vi "rad_Modify and Deploy RT-INI.vi"(5 "password":string, 7 "user (admin)":string="admin", 8 "error in (no error)":errorcluster, 9 "Run at Startup?":bool, 10 "Target settings":T1={"Hostname"="", "Serial number"="", "Product name"="", "Product code"=0, "System status"="", "Credential type"=enum."None/Unlocked", "User added?"=FALSE, "Primary NIC"={"MAC address"="", "IP Address Request Mode"=2, "IP address"="", "Subnet mask"="", "Gateway"="", "DNS server"=""}, "Real-Time CPU?"=FALSE} {"Primary NIC"."IP Address Request Mode" items=["Static"=1, "DHCP/Link-Local"=2, "Link-Local Only"=4, "DHCP Only"=8]}, 11 "temp folder":path) -> (0 "error out":errorcluster)   [LabVIEW 2018]
uses:
  Targets/TypeDefs/rad_Target Information.ctl
  Targets/TypeDefs/rad_Target Network Settings.ctl
  rad_Globals.vi
  <vilib>/Utility/config.llb/Write Key (Boolean).vi
  <vilib>/nisyscfg/Save Changes (Hardware).vi
  <vilib>/nisyscfg/Close (Hardware).vi
  <vilib>/nisyscfg/Close (System).vi
  <vilib>/Utility/config.llb/NI_LVConfig.lvlib
  <resource>/objmgr/motionsysapi.rc
  <resource>/objmgr/nisysapi.rc
  <vilib>/nisyscfg/nisyscfg.lvlib
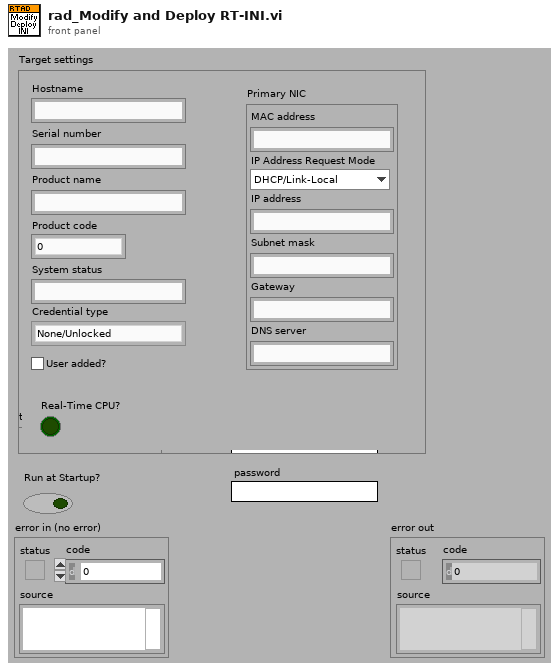
[diagram p1: front panel]
types:
  T1 = typedef "rad_Target Information.ctl" = cluster{"Hostname":string, "Serial number":string, "Product name":string, "Product code":i32, "System status":string, "Credential type":enum16{"None/Unlocked", "FTP Password", "NIAuth Credentials"}, "User added?":bool, "Primary NIC":T2, "Real-Time CPU?":bool}
  T2 = typedef "rad_Target Network Settings.ctl" = cluster{"MAC address":string, "IP Address Request Mode":i32, "IP address":string, "Subnet mask":string, "Gateway":string, "DNS server":string}
  T3 = enum16{"None/Unlocked", "FTP Password", "NIAuth Credentials"}
  T4 = typedef "NI_LVConfig.lvlib/Config Data RefNum.ctl" = refnum<k1>
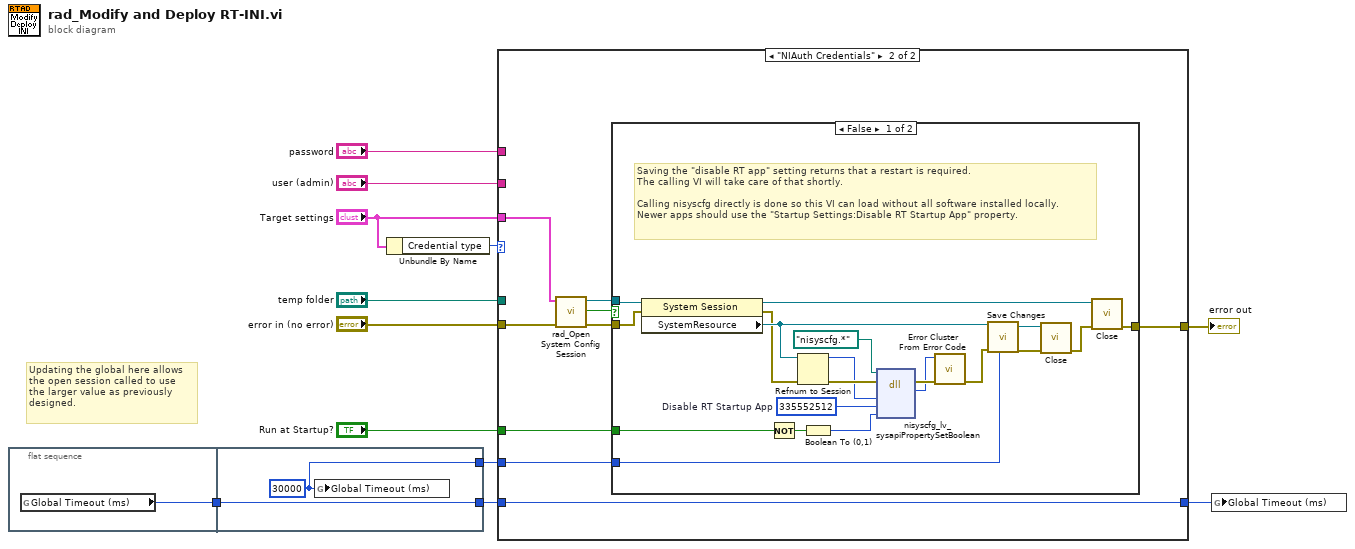
[diagram p0: block diagram]
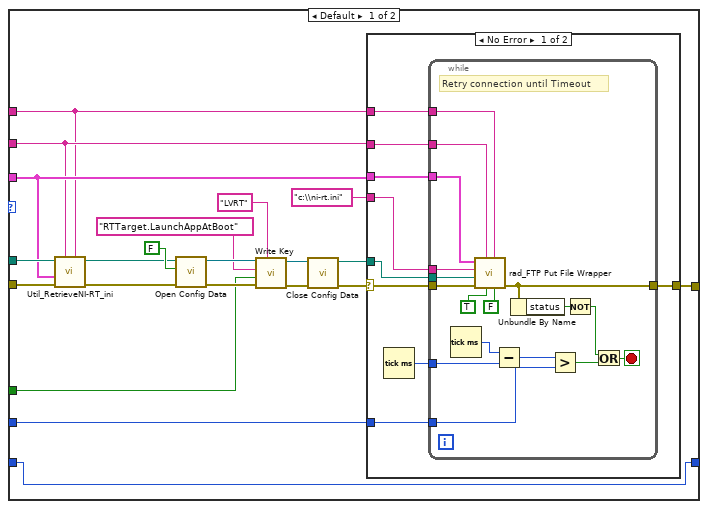
[diagram p2: hidden frame]
diagram:
  # "Updating the global here allows\nthe open session called to use\nthe larger value as previously\ndesigned."
  n1 = flat-sequence {
    tunnel: [w13] -> w4
    tunnel: [w15] -> w2
    tunnel: w4 -> [w15]
    tunnel: [w14] -> w3
    frame #0 {
      n2 = global read "rad_Globals.vi" "Global Timeout (ms)"() -> (w13:u32)
    }
    frame #1 {
      w14 = u32 30000 ("Global Timeout (ms)")
      n3 = global write "rad_Globals.vi" "Global Timeout (ms)"(w14) -> ()
    }
  }
  n4 = Unbundle By Name("Target settings") -> ("Credential type"=w5:T3)
  n5 = case shown="\"NIAuth Credentials\"" w5 {
    tunnel: "Run at Startup?" -> [w31 w66]
    tunnel: w3 -> [w28 w65]
    tunnel: "user (admin)" -> [w18 _]
    tunnel: "password" -> [w17 _]
    tunnel: [w24 w67] -> w9
    tunnel: "temp folder" -> [w23 _]
    tunnel: "error in (no error)" -> [w21 w71]
    tunnel: "Target settings" -> [w19 w72]
    tunnel: w2 -> [w16 w64]
    tunnel: [w16 w64] -> w1
    frame Default {
      n6 = call "Util_RetrieveNI-RT_ini.vi"("password"=w17, "user (admin)"=w18, "error in"=w21, "Target settings"=w19, "temp folder"=w23) -> ("error out"=w20:errorcluster, "Ini File Path"=w22:path)  [unwired: 5 in]
      n7 = call <vilib>:"Open Config Data.vi"("error in (no error)"=w20, "create file if necessary (T)"=FALSE, "configuration file path"=w22) -> ("error out"=w35:errorcluster, "refnum"=w34:T4)  [unwired: 6 in, 1 out]
      n8 = call-poly <vilib>:"Write Key.vi"("section"="LVRT", "error in (no error)"=w35, "value"=w31, "key"="RTTarget.LaunchAppAtBoot", "refnum"=w34) -> ("error out"=w29:errorcluster, "refnum out"=w30:T4)  [unwired: 4 in, 1 out]
      n9 = call <vilib>:"Close Config Data.vi"("error in (no error)"=w29, "refnum"=w30) -> ("error out"=w27:errorcluster, "file path"=w25:path)  [unwired: 8 in]
      n10 = case shown="No Error" w27 {
        selector: w27 -> [w44 w63]
        tunnel: [w43 w63] -> w24
        tunnel: w28 -> [w42 _]
        tunnel: "c:\\ni-rt.ini" ("remote path") -> [w41 _]
        tunnel: w25 -> [w40 _]
        tunnel: w19 -> [w39 _]
        tunnel: w18 -> [w38 _]
        tunnel: w17 -> [w37 _]
        frame No Error {
          n11 = Tick Count (ms)() -> (millisecond timer value=w45:u32)
          n12 = while {
            tunnel: w44 -> [w55]
            tunnel: w45 -> [w61]
            tunnel: [w54] -> w43
            tunnel: w42 -> [w53]
            tunnel: w41 -> [w52]
            tunnel: w40 -> [w51]
            tunnel: w39 -> [w50]
            tunnel: w38 -> [w49]
            tunnel: w37 -> [w48]
            stop <- w57 stop-if-true
            # "Retry connection until Timeout"
            n13 = Tick Count (ms)() -> (millisecond timer value=w62:u32)
            n14 = call "rad_FTP Put File Wrapper.vi"("active (F)"=FALSE ("active (T)"), "password"=w48, "binary (T)"=TRUE ("binary (F)"), "user (admin)"=w49, "error in (no error)"=w55, "local path"=w51, "remote path"=w52, "Target settings"=w50) -> ("error out"=w54:errorcluster)  [unwired: 3 in]
            n15 = Subtract(x=w62, y=w61) -> (x-y=w60:u32)
            n16 = Unbundle By Name(w54) -> ("status"=w56:bool)
            n17 = Greater?(x=w60, y=w53) -> (0:w58:bool)
            n18 = Not(x=w56) -> (.not. x?=w59:bool)
            n19 = Or(x=w59, y=w58) -> (x .or. y?=w57:bool)
          }
        }
        frame Error {
        }
      }
    }
    frame "NIAuth Credentials" {
      n20 = call "rad_Open System Config Session.vi"("error in (no error)"=w71, "Target settings"=w72) -> ("error out"=w68:errorcluster, "Cancelled"=w70:bool, "Session out"=w69:refnum<k21>)  [unwired: 6 in, 1 out]
      n21 = case shown="False" w70 {
        tunnel: w69 -> [w92 _]
        tunnel: w68 -> [w91 w93]
        tunnel: [w85 w93] -> w67
        tunnel: w66 -> [w90 _]
        tunnel: w65 -> [w84 _]
        frame False {
          w79 = u32 335552512  # Disable RT Startup App
          # "Saving the \"disable RT app\" setting returns that a restart is required.\nThe calling VI will take care of that shortly.\n\nCalling nisyscfg directly is done so this VI can load without all software installed locally.\nNewer apps should use the \"Startup Settings:Disable RT Startup App\" property."
          n22 = property class="System Session"(reference=w92, error in=w91) -> (reference out=w89:refnum<k21>, error out=w76:errorcluster, "SystemResource"=w77:refnum<k20>)
          n23 = Not(x=w90) -> (.not. x?=w74:bool)
          n24 = Refnum to Session(4:w76, 7:w77) -> (0:w83:errorcluster, 3:w78:u64)
          n25 = Boolean To (0,1)(Boolean=w74) -> (0, 1=w73:i16)
          n26 = dll-call lib="nisyscfg.dll" fn="nisyscfg_lv_sysapiPropertySetBoolean"(path in=path "nisyscfg.*", error in=w83, "resource"=w78, "attribute"=w79, "value"=w73) -> (error out=w82:errorcluster, "status"=w80:i32)  [unwired: 4 in, 1 out]
          n27 = call <vilib>:"Error Cluster From Error Code.vi"("error in (no error)"=w82, "error code (0)"=w80) -> ("error out"=w75:errorcluster)  [unwired: 2 in, 5 out]
          n28 = call-poly <vilib>:"Save Changes.vi"("Remote Timeout (300,000 ms)"=w84, "error in (no error)"=w75, "Resource in"=w77) -> ("error out"=w87:errorcluster, "Resource out"=w88:refnum<k20>)  [unwired: 5 in, 2 out]
          n29 = call-poly <vilib>:"Close.vi"("error in (no error)"=w87, "Resource in"=w88) -> ("error out"=w86:errorcluster)  [unwired: 9 in]
          n30 = call-poly <vilib>:"Close.vi"("error in (no error)"=w86, "Session in"=w89) -> ("error out"=w85:errorcluster)  [unwired: 9 in]
        }
        frame True {
        }
      }
    }
  }
  "error out" <- w9
  n31 = global write "rad_Globals.vi" "Global Timeout (ms)"(w1) -> ()
